vi "trigger_rising_edge.vi"(11 "input":bool) -> (3 "rising":bool)   [LabVIEW 2014]
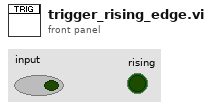
[diagram p1: front panel]
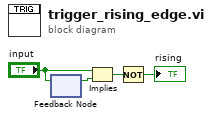
[diagram p0: block diagram]
diagram:
  n1 = feedback-in #1("input") -> ()
  n2 = feedback #1() -> (w2:bool)  [unwired: 1 in]
  n3 = Implies(1:w2, 2:"input") -> (0:w4:bool)
  n4 = Not(x=w4) -> (.not. x?=→"rising":bool)
